vi "CIPC CAN FIFO.vi"() -> (3 "CIF_CIPC_CAN.lvclass":refnum<class "CIF_CIPC_CAN.lvclass">)   [LabVIEW 2021, in "CIF_CIPC_CAN.lvclass"]
uses:
  CIF_CIPC_CAN.lvclass
  CIF_CIPC_CAN.lvclass/CIF_CIPC_CAN.ctl
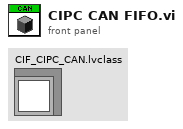
[diagram p1: front panel]
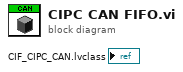
[diagram p0: block diagram]
diagram:
